vi "DAC_nextEnabledChannel.vi"(10 "DAC channel enable":T1={"ch0"=TRUE, "ch1"=TRUE, "ch2"=TRUE, "ch3"=TRUE, "ch4"=TRUE, "ch5"=TRUE, "ch6"=TRUE}, 11 "channel index in":u16 max=7 step=1) -> (3 "nextEnabledChannelIndex":u16)   [LabVIEW 2010]
uses:
  common_typedefs/DAC_channel_enable_cluster.ctl
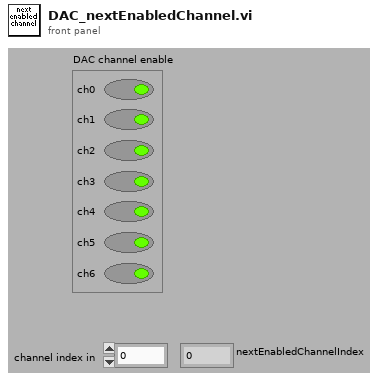
[diagram p1: front panel]
types:
  T1 = typedef "DAC_channel_enable_cluster.ctl" = cluster{"ch0":bool, "ch1":bool, "ch2":bool, "ch3":bool, "ch4":bool, "ch5":bool, "ch6":bool}
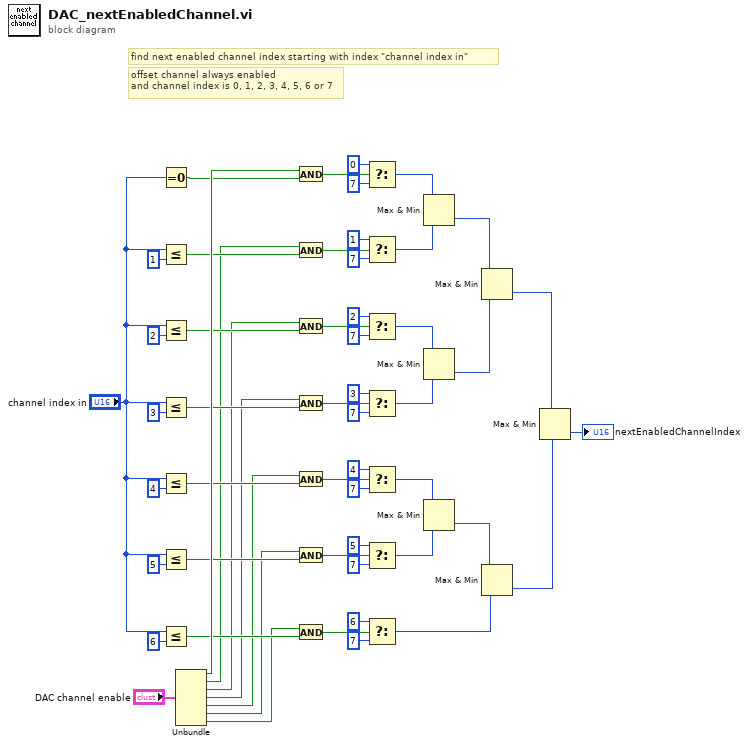
[diagram p0: block diagram]
diagram:
  # "offset channel always enabled\nand channel index is 0, 1, 2, 3, 4, 5, 6 or 7"
  # "find next enabled channel index starting with index \"channel index in\""
  n1 = Equal To 0?(x="channel index in") -> (x = 0?=w4:bool)
  n2 = Less Or Equal?(x="channel index in", y=u16 1) -> (x <= y?=w49:bool)
  n3 = Less Or Equal?(x="channel index in", y=u16 2) -> (x <= y?=w48:bool)
  n4 = Less Or Equal?(x="channel index in", y=u16 3) -> (x <= y?=w47:bool)
  n5 = Less Or Equal?(x="channel index in", y=u16 4) -> (x <= y?=w46:bool)
  n6 = Less Or Equal?(x="channel index in", y=u16 5) -> (x <= y?=w44:bool)
  n7 = Less Or Equal?(x="channel index in", y=u16 6) -> (x <= y?=w45:bool)
  n8 = Unbundle("DAC channel enable") -> ("ch0"=w50:bool, "ch1"=w11:bool, "ch2"=w10:bool, "ch3"=w9:bool, "ch4"=w8:bool, "ch5"=w7:bool, "ch6"=w6:bool)
  n9 = And(x=w50, y=w4) -> (x .and. y?=w43:bool)
  n10 = And(x=w11, y=w49) -> (x .and. y?=w42:bool)
  n11 = And(x=w10, y=w48) -> (x .and. y?=w41:bool)
  n12 = And(x=w9, y=w47) -> (x .and. y?=w40:bool)
  n13 = And(x=w8, y=w46) -> (x .and. y?=w39:bool)
  n14 = And(x=w7, y=w44) -> (x .and. y?=w38:bool)
  n15 = And(x=w6, y=w45) -> (x .and. y?=w37:bool)
  n16 = Select(t=u16 0, s=w43, f=u16 7) -> (s? t:f=w36:u16)
  n17 = Select(t=u16 1, s=w42, f=u16 7) -> (s? t:f=w35:u16)
  n18 = Select(t=u16 2, s=w41, f=u16 7) -> (s? t:f=w34:u16)
  n19 = Select(t=u16 3, s=w40, f=u16 7) -> (s? t:f=w33:u16)
  n20 = Select(t=u16 4, s=w39, f=u16 7) -> (s? t:f=w32:u16)
  n21 = Select(t=u16 5, s=w38, f=u16 7) -> (s? t:f=w31:u16)
  n22 = Select(t=u16 6, s=w37, f=u16 7) -> (s? t:f=w2:u16)
  n23 = Max & Min(x=w36, y=w35) -> (min(x,y)=w30:u16)  [unwired: 1 out]
  n24 = Max & Min(x=w34, y=w33) -> (min(x,y)=w29:u16)  [unwired: 1 out]
  n25 = Max & Min(x=w32, y=w31) -> (min(x,y)=w28:u16)  [unwired: 1 out]
  n26 = Max & Min(x=w30, y=w29) -> (min(x,y)=w27:u16)  [unwired: 1 out]
  n27 = Max & Min(x=w28, y=w2) -> (min(x,y)=w26:u16)  [unwired: 1 out]
  n28 = Max & Min(x=w27, y=w26) -> (min(x,y)=→"nextEnabledChannelIndex":u16)  [unwired: 1 out]
